vi "FIB trapezoidal mill PXIe-6124.vi"(6 "Machine Type":u8(ring) items=["Feiss", "NVision", "Jeiss"], 7 "COM port":refnum<visa-resource-name>="COM1", 8 "Milling para":T1={"X resolution"=4096, "Z resolution"=125001, "X offset (um)"=0.0, "Z offset (um)"=0.0, "X center (um)"=0.0, "Z center (um)"=0.0, "X size (um)"=250.0, "Z size (um)"=250.0, "UL-Ang"=90.0, "UR-Ang"=90.0, "Line milling time (s)"=5.0, "Z-step (nm)"=2.0, "Lines auto pause"=1, "Auto pause"=FALSE, "Mill from Bottom"=FALSE, "FIB FOV (um)"=500.0, "Auto Profile"=FALSE, "Mill start from Last"=FALSE, "FIB PID on"=FALSE, "FIB PID reset"=TRUE, "FIB PID measured"=0, "FIB PID target"=0.0, "FIB PID target slope"=0.0, "FIB PID P"=0.001, "FIB PID I"=0.01, "FIB PID D"=0.0, "Emission (uA)"=1.36, "Suppressor (V)"=50.0, "Auto reheat"=FALSE} caption="Milling Parameters" {"Suppressor (V)" step=0.1 format="%.1g"; "Emission (uA)" step=0.1 format="%.2g"; "FIB PID measured" items=["Spec.", "B.D. 1", "B.D. 2", "Mill", "Spec. +"]; "FIB PID target slope" min=-1 max=1 step=0.1; "UR-Ang" format="%.2f"; "UL-Ang" format="%.2f"; "Z offset (um)" step=0.02 format="%.3g"; "X offset (um)" step=1 format="%.3g"; "FIB FOV (um)" format="%.3g"; "Line milling time (s)" format="%.1f"; "Z center (um)" format="%#.3g"; "X center (um)" format="%#.3g"}, 9 "Options":cluster{"Flip x":bool, "Flip z":bool}={"Flip x"=TRUE, "Flip z"=TRUE}, 10 "FIB Scan Parameters":T3={"X resolution"=512, "Z resolution"=512, "X center"=0.0, "Z center"=0.0, "X size (V)"=20.0, "Z size (V)"=20.0, "Frame line rampdown ratio"=-0.1, "Scan rate (Hz)"=2000000, "Oversampling"=2} {"Z size (V)" min=0.0 max=20.0; "X size (V)" min=0.0 max=20.0; "Frame line rampdown ratio" min=-1.0 max=1.0 step=0.05 format="%.2g"; "Scan rate (Hz)" max=4000000 format="%#.6p"; "Z resolution" max=2048; "X resolution" max=2048}, 11 "HW Config":T4={"FIB X coil"="FIB/ao0", "FIB Y coil"="FIB/ao1", "Beam blank"="FIB/port0/line0", "Ext scan"="FIB/port0/line1", "Detector"="FIB/ai0", "Post #1up"="Log/ao0", "Post #1down"="Log/ao1", "Post #2up"="Log/ao2", "Post #2down"="Log/ao3"}) -> (0 "error out":errorcluster, 1 "post-pause lines":u16, 2 "Total progress":u8(slide) scale=0.0..100.0, 3 "Line progress":u8(slide) scale=0.0..100.0)   [LabVIEW 2018]
uses:
  <vilib>/DAQmx/write.llb/DAQmx Write (Analog 2D DBL NChan NSamp).vi
  <vilib>/DAQmx/write.llb/DAQmx Write (Analog 1D DBL 1Chan NSamp).vi
  <vilib>/Analysis/baseanly.llb/Mean (DBL).vi
  <vilib>/DAQmx/write.llb/DAQmx Write (Analog DBL 1Chan 1Samp).vi
  <vilib>/DAQmx/write.llb/DAQmx Write (Analog 1D DBL NChan 1Samp).vi
  <vilib>/DAQmx/create/channels.llb/DAQmx Create Channel (AO-Voltage-Basic).vi
  <vilib>/DAQmx/configure/timing.llb/DAQmx Timing (Sample Clock).vi
  <vilib>/DAQmx/miscellaneous.llb/DAQmx Fill In Error Info.vi
  <vilib>/measure/madcrms.llb/Basic Averaged DC-RMS for 1 Chan.vi
  <vilib>/Analysis/NI_AALBase.lvlib
  <vilib>/measure/NI_MAPro.lvlib
panel:
  in  "Api":refnum<k7>(container)
  out "FIB PID measured":u8
  out "FIB PID on offset":dbl
  out "FIB PID target slope":sgl
  out "FIB PID feedback mean":dbl
  out "FIB PID FB array":dbl[](array[numeric])
  out "Beam blanked":bool=TRUE
  out "FIB PID D":sgl
  out "FIB PID I":sgl
  out "FIB PID P":sgl
  out "FIB PID target":sgl
  out "FIB PID reset":bool
  out "FIB PID on":bool
  out "FIB PID feedback":dbl
  out "UR-Ang":sgl=90.0
  out "UL-Ang":sgl=90.0
  in  "FIB bit size (nm)":dbl
  out "X offset":sgl
  out "Y offset":sgl
  in  "Sweep enabled":bool
  in  "Focus (V)":dbl min=-10.0 max=10.0 step=0.1 format="%.3g"
  in  "Imbalance (V)":dbl min=-10.0 max=10.0 step=0.1 format="%.3f"
  in  "Sweep direction":bool
  in  "Angle (V)":dbl min=-10.0 max=10.0 step=0.1 format="%.3g"
  in  "Position (V)":dbl min=-10.0 max=10.0 step=0.1 format="%.3g"
  in  "Level #":u8
  in  "Sweep #":u8=1 min=1
  out "Post #2down":tag="PXI1Slot2/ao3"
  out "Post #2up":tag="PXI1Slot2/ao2"
  out "Post #1down":tag="PXI1Slot2/ao1"
  out "Post #1up":tag="PXI1Slot2/ao0"
  out "Milling mode":T2(ring)=enum."SEM + FIB"
  out "Z voltage RT":dbl
  out "Ext scan":tag="PXI1Slot4/port0/line1"
  out "FIB Y coil":tag="PXI1Slot4/ao1"
  out "FIB X coil":tag="PXI1Slot4/ao0"
  out "Mill from Bottom":bool
  out "Line Paused":bool
  in  "Resume":bool
  in  "Manual pause":bool
  out "Auto pause":bool
  out "Line milling time (s)":sgl=10.0
  out "Lines auto pause":u16=1
  out "Y size":sgl=1.0
  out "X size":sgl=1.0
  out "Y center":sgl
  out "X center":sgl
  out "Y resolution":u32=100
  out "X resolution":u32=16384
  in  "Stop":bool
  out "Beam blank":tag="PXI1Slot4/port0/line0"
  # "% of"
  # "th line"
  # "%"
  # "Direction"
  # "Start\nfrom"
  # "<"
  # "Scan coils"
  # "Flip"
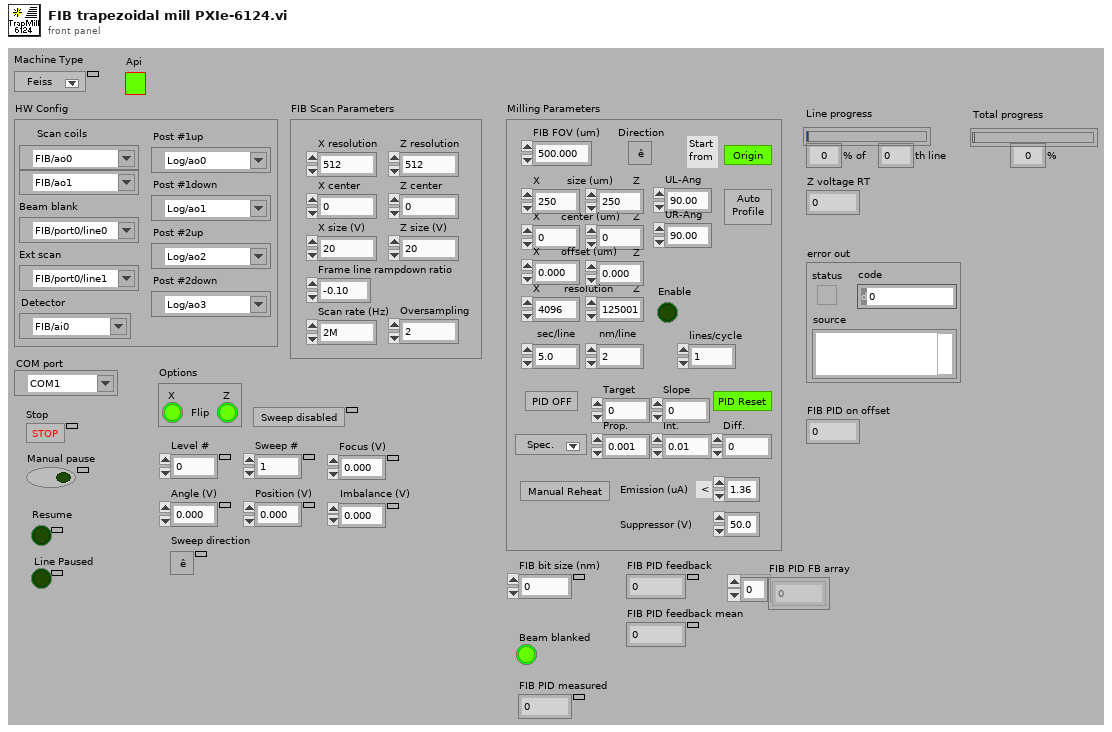
[diagram p1: front panel]
types:
  T1 = cluster{"X resolution":u32, "Z resolution":u32, "X offset (um)":sgl, "Z offset (um)":sgl, "X center (um)":sgl, "Z center (um)":sgl, "X size (um)":sgl, "Z size (um)":sgl, "UL-Ang":sgl, "UR-Ang":sgl, "Line milling time (s)":sgl, "Z-step (nm)":dbl, "Lines auto pause":u16, "Auto pause":bool, "Mill from Bottom":bool, "FIB FOV (um)":sgl, "Auto Profile":bool, "Mill start from Last":bool, "FIB PID on":bool, "FIB PID reset":bool, "FIB PID measured":u8, "FIB PID target":sgl, "FIB PID target slope":sgl, "FIB PID P":sgl, "FIB PID I":sgl, "FIB PID D":sgl, "Emission (uA)":dbl, "Suppressor (V)":sgl, "Auto reheat":bool}
  T2 = enum16{"SEM", "FIB", "Milling", "SEM + FIB", "Mill + SEM", "SEM Drift Correction", "FIB Drift Correction", "No Beam", "External", "External + SEM"}
  T3 = cluster{"X resolution":u32, "Z resolution":u32, "X center":dbl, "Z center":dbl, "X size (V)":dbl, "Z size (V)":dbl, "Frame line rampdown ratio":dbl, "Scan rate (Hz)":u32, "Oversampling":u16}
  T4 = cluster{"FIB X coil":tag, "FIB Y coil":tag, "Beam blank":tag, "Ext scan":tag, "Detector":tag, "Post #1up":tag, "Post #1down":tag, "Post #2up":tag, "Post #2down":tag}
  T5 = enum16{"SEM", "FIB", "Mill", "SEM + FIB", "Mill + SEM", "Drift SEM", "Drift FIB", "None", "Ext", "Ext + SEM"}
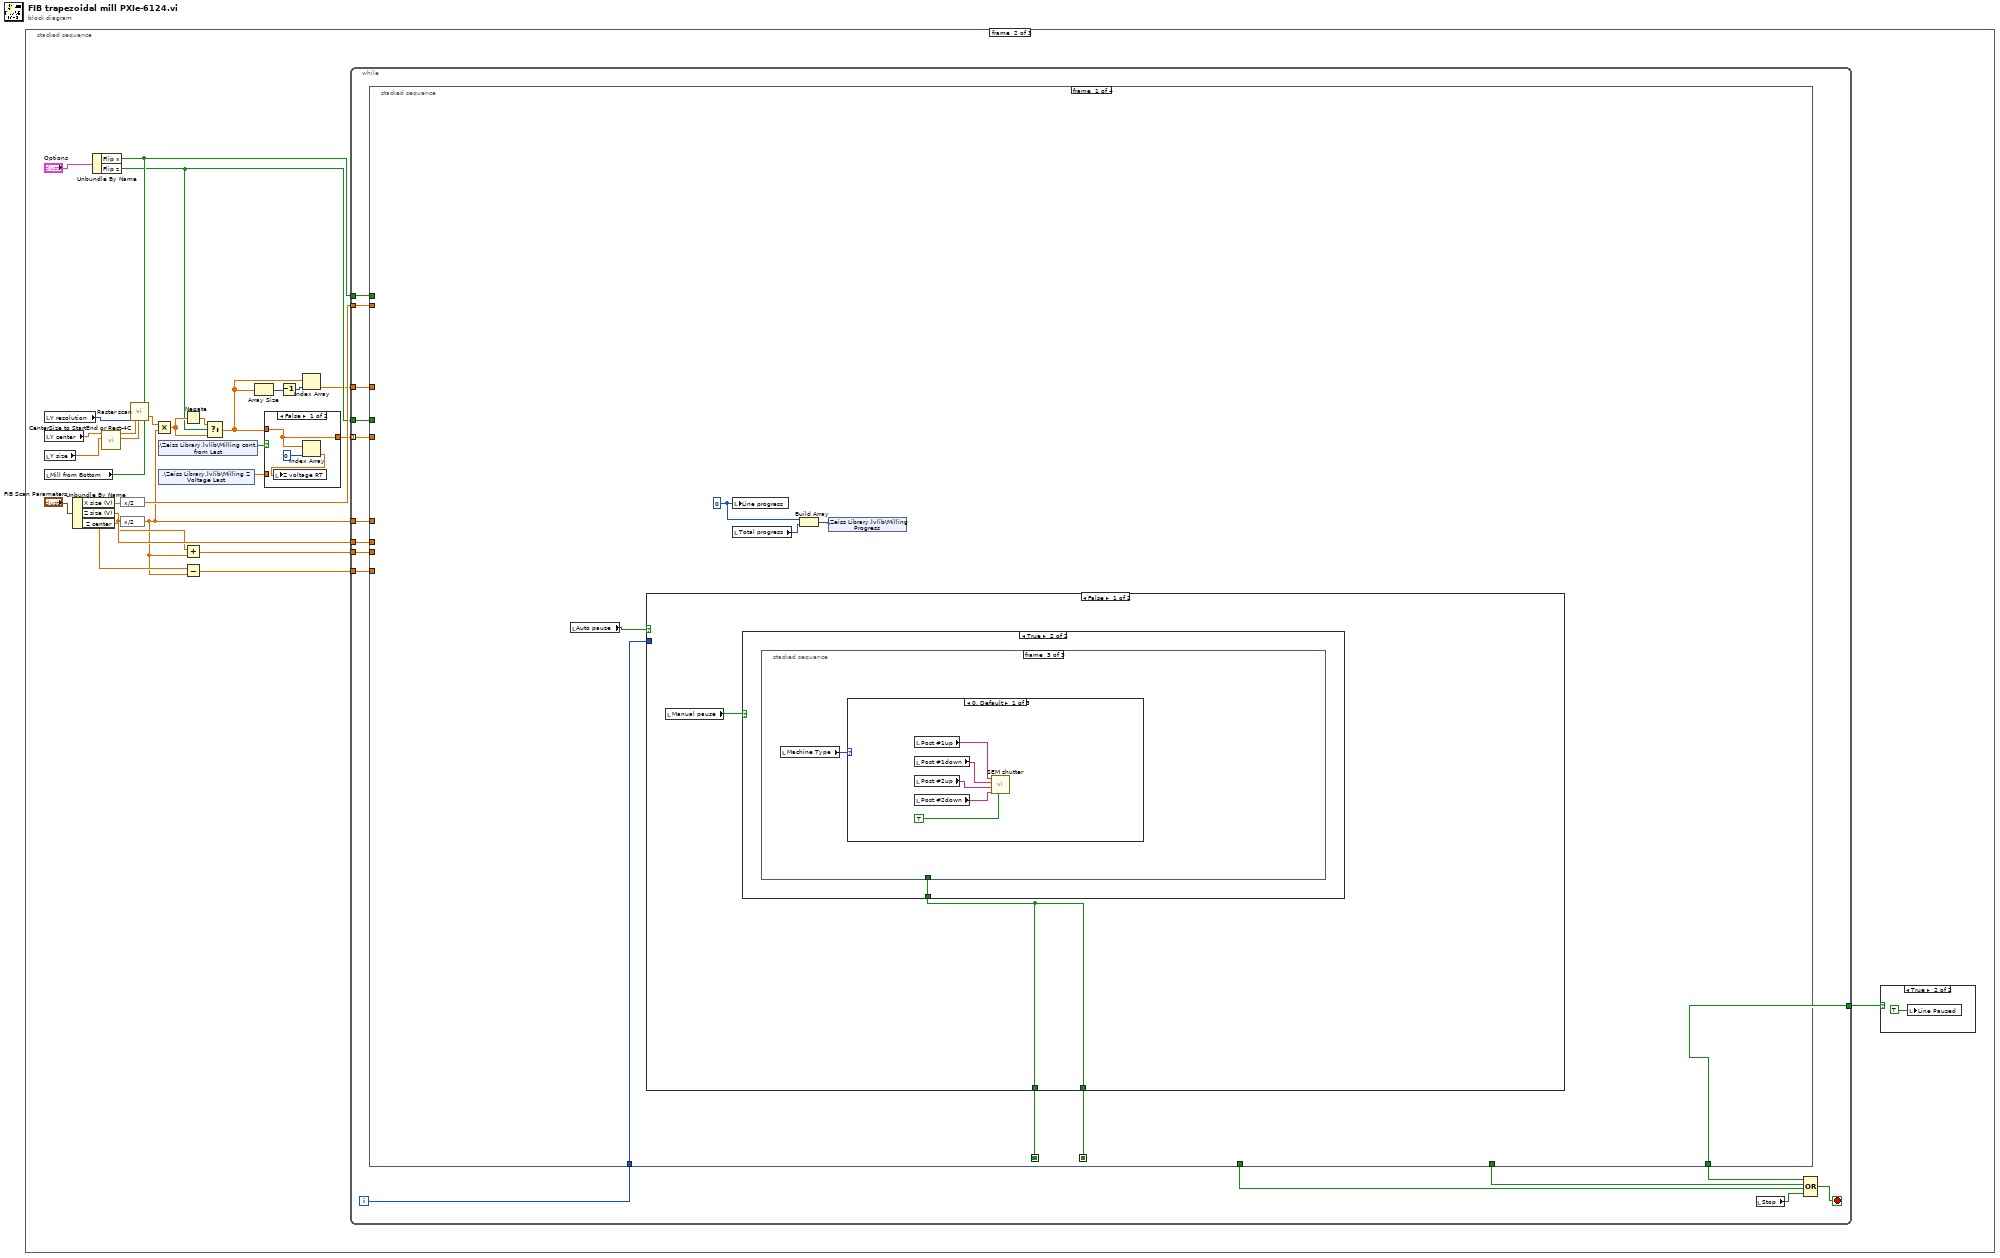
[diagram p0: block diagram]
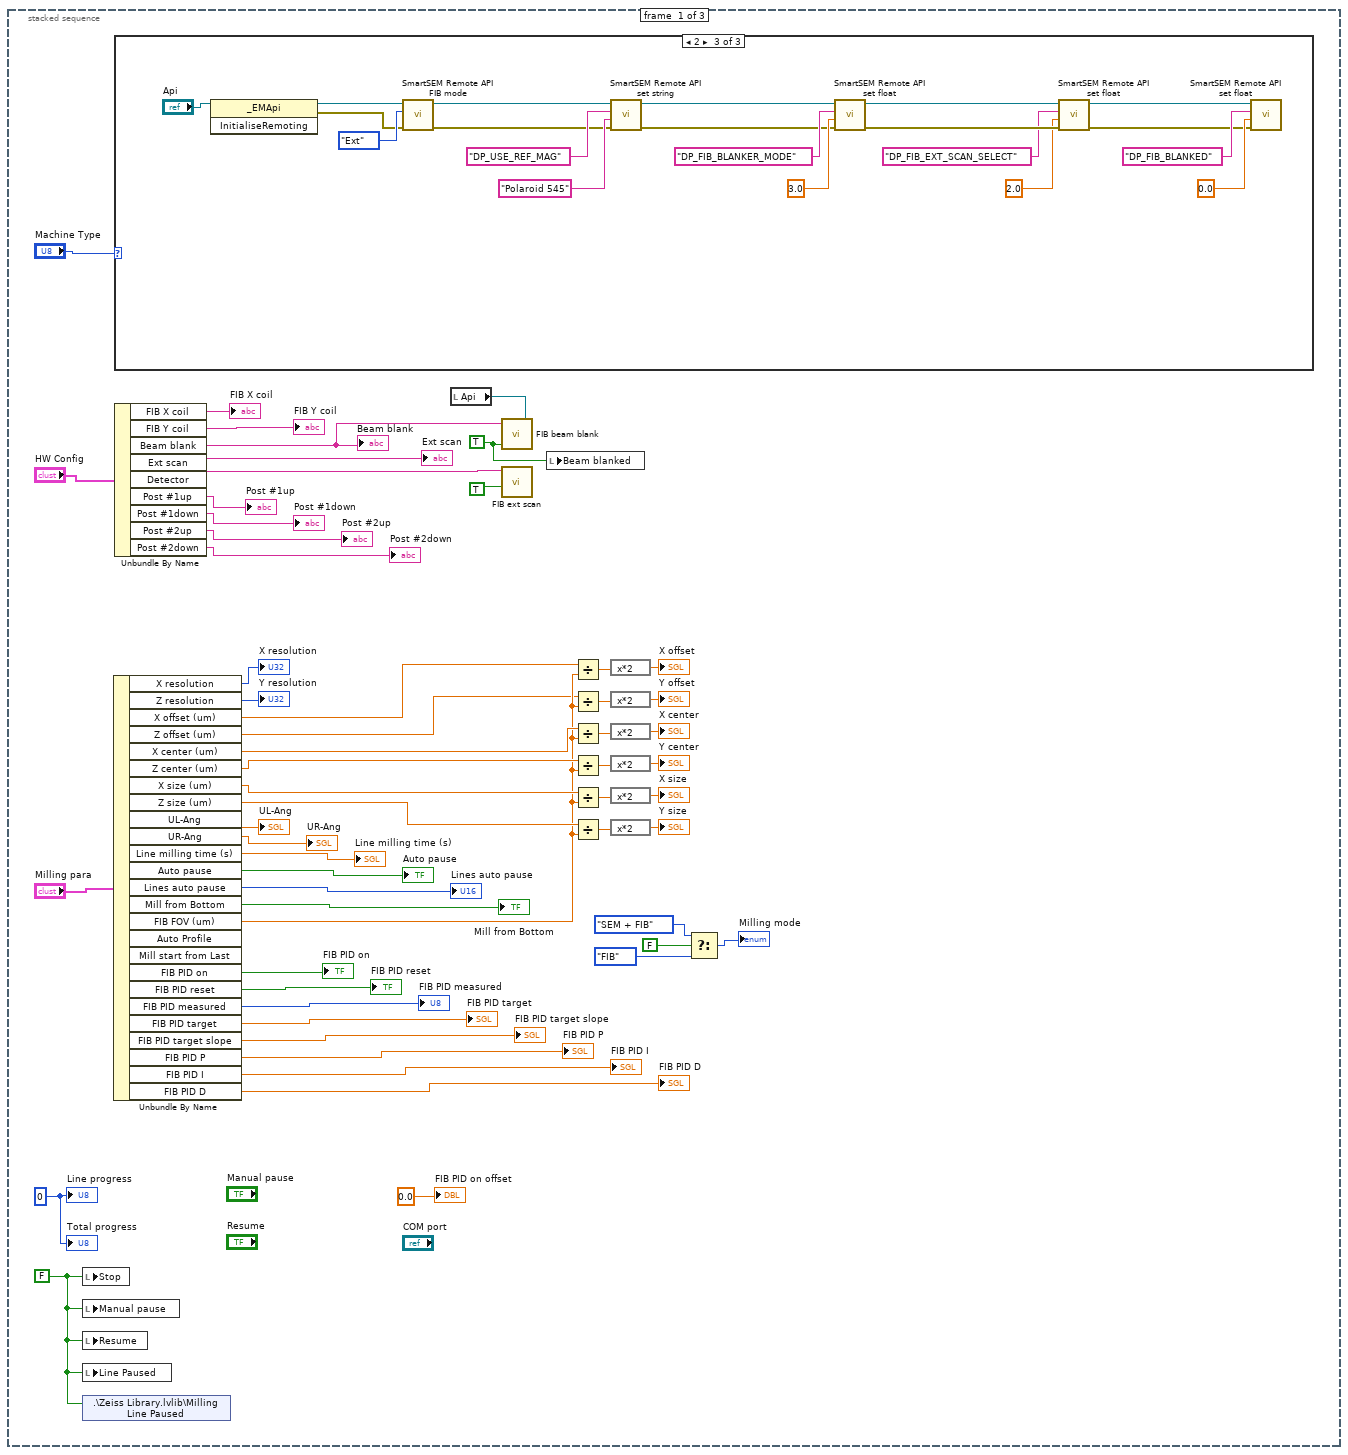
[diagram p2: hidden frame]
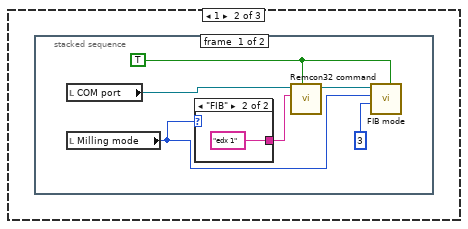
[diagram p4: hidden frame]
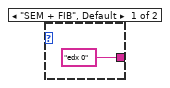
[diagram p5: hidden frame]
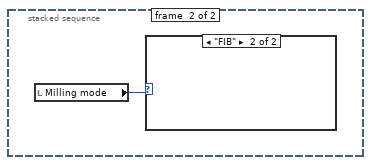
[diagram p6: hidden frame]
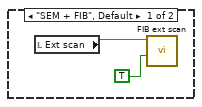
[diagram p7: hidden frame]
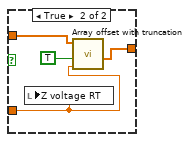
[diagram p8: hidden frame]
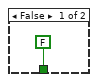
[diagram p10: hidden frame]
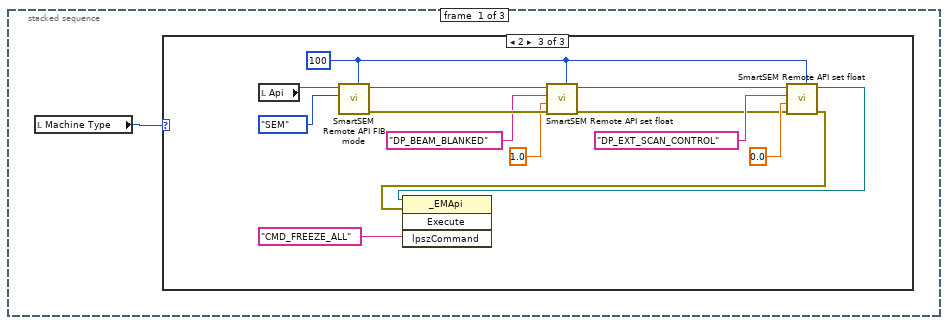
[diagram p11: hidden frame]
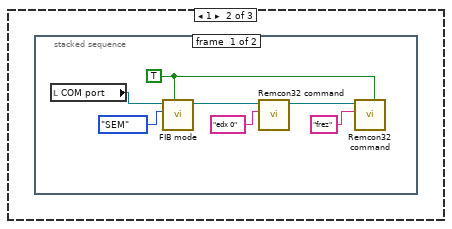
[diagram p13: hidden frame]
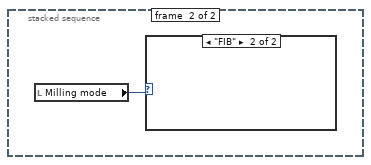
[diagram p14: hidden frame]
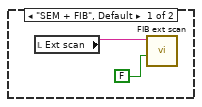
[diagram p15: hidden frame]
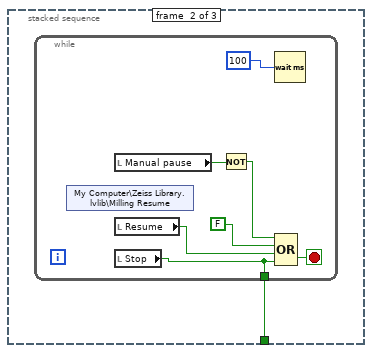
[diagram p16: hidden frame]
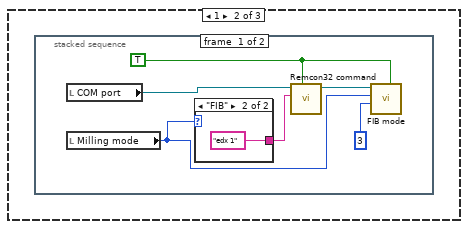
[diagram p17: hidden frame]
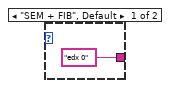
[diagram p18: hidden frame]
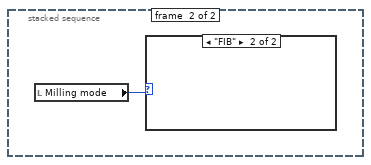
[diagram p19: hidden frame]
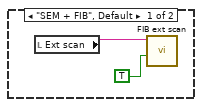
[diagram p20: hidden frame]
diagram:
  n1 = stacked-sequence {
    frame #0 {
      w7 = TRUE ("Beam blanked")
      w46 = FALSE ("Stop")
      w56 = u8 0 ("Milling progress")
      n2 = local write "Stop"(w46) -> ()
      n3 = local write "Manual pause"(w46) -> ()
      n4 = local write "Resume"(w46) -> ()
      n5 = local write "Line Paused"(w46) -> ()
      n6 = shared-variable ".\\Zeiss Library.lvlib\\Milling Line Paused"(w46) -> ()  [unwired: 1 in, 1 out]
      n7 = Unbundle By Name("Milling para") -> ("X resolution"=→"X resolution":u32, "Z resolution"=→"Y resolution":u32, "X offset (um)"=w22:sgl, "Z offset (um)"=w21:sgl, "X center (um)"=w27:sgl, "Z center (um)"=w26:sgl, "X size (um)"=w37:sgl, "Z size (um)"=w33:sgl, "UL-Ang"=→"UL-Ang":sgl, "UR-Ang"=→"UR-Ang":sgl, "Line milling time (s)"=→"Line milling time (s)":sgl, "Auto pause"=→"Auto pause":bool, "Lines auto pause"=→"Lines auto pause":u16, "Mill from Bottom"=→"Mill from Bottom":bool, "FIB FOV (um)"=w23:sgl, "FIB PID on"=→"FIB PID on":bool, "FIB PID reset"=→"FIB PID reset":bool, "FIB PID measured"=→"FIB PID measured":u8, "FIB PID target"=→"FIB PID target":sgl, "FIB PID target slope"=→"FIB PID target slope":sgl, "FIB PID P"=→"FIB PID P":sgl, "FIB PID I"=→"FIB PID I":sgl, "FIB PID D"=→"FIB PID D":sgl)  [unwired: 2 out]
      n8 = case shown="2" "Machine Type" {
        frame 0, Default {
        }
        frame 1 {
          n9 = stacked-sequence {
            frame #0 {
              w59 = TRUE ("Initialization")
              n10 = local read "COM port"() -> (w61:refnum<visa-resource-name>)
              n11 = local read "Milling mode"() -> (w57:T2)
              n12 = case shown="\"FIB\"" w57 {
                tunnel: ["edx 0" ("SEM command") "edx 1" ("SEM command")] -> w58
                frame "SEM + FIB", Default {
                }
                frame "FIB" {
                }
              }
              n13 = call "Remcon32 command.vi"("Initialization"=w59, "SEM command"=w58, "COM port in"=w61) -> ("COM port out"=w60:refnum<visa-resource-name>)  [unwired: 5 in, 3 out]
              n14 = call "FIB mode.vi"("Close session"=w59, "Iterations"=u32 3, "FIB mode"=w57, "COM port in"=w60) -> ()  [unwired: 6 in, 2 out]
            }
            frame #1 {
              n15 = local read "Milling mode"() -> (w65:T2)
              n16 = case shown="\"FIB\"" w65 {
                frame "SEM + FIB", Default {
                  n17 = local read "Ext scan"() -> (w66:tag)
                  n18 = call "FIB ext scan.vi"("Ext on"=TRUE ("data"), "FIB Ext Scan"=w66) -> ()  [unwired: 9 in, 1 out]
                }
                frame "FIB" {
                }
              }
            }
          }
        }
        frame 2 {
          n19 = invoke class="_EMApi" method="InitialiseRemoting"(reference="Api") -> (reference out=w85:refnum<k7>, error out=w84:errorcluster)  [unwired: 2 in, 1 out]
          n20 = call "SmartSEM Remote API FIB mode.vi"("error in"=w84, "FIB mode"=T5."Ext", "Api"=w85) -> ("error out"=w68:errorcluster, "Api out"=w71:refnum<k7>)  [unwired: 7 in]
          n21 = call "SmartSEM Remote API set string.vi"("error in"=w68, "vValue"="Polaroid 545" ("lpszParam"), "lpszParam"="DP_USE_REF_MAG", "Api"=w71) -> ("error out"=w69:errorcluster, "Api out"=w70:refnum<k7>)  [unwired: 6 in]
          n22 = call "SmartSEM Remote API set float.vi"("error in"=w69, "vValue"=sgl 3.0, "lpszParam"="DP_FIB_BLANKER_MODE", "Api"=w70) -> ("error out"=w78:errorcluster, "Api out"=w79:refnum<k7>)  [unwired: 6 in]
          n23 = call "SmartSEM Remote API set float.vi"("error in"=w78, "vValue"=sgl 2.0, "lpszParam"="DP_FIB_EXT_SCAN_SELECT" ("lpszCommand"), "Api"=w79) -> ("error out"=w72:errorcluster, "Api out"=w73:refnum<k7>)  [unwired: 6 in]
          n24 = call "SmartSEM Remote API set float.vi"("error in"=w72, "vValue"=sgl 0.0, "lpszParam"="DP_FIB_BLANKED", "Api"=w73) -> ()  [unwired: 6 in, 2 out]
        }
      }
      n25 = Unbundle By Name("HW Config") -> ("FIB X coil"=→"FIB X coil":tag, "FIB Y coil"=→"FIB Y coil":tag, "Beam blank"=w43:tag, "Ext scan"=w44:tag, "Post #1up"=→"Post #1up":tag, "Post #1down"=→"Post #1down":tag, "Post #2up"=→"Post #2up":tag, "Post #2down"=→"Post #2down":tag)  [unwired: 1 out]
      "Beam blank" <- w43
      "Ext scan" <- w44
      n26 = local read "Api"() -> (w2:refnum<k7>)
      n27 = call "FIB beam blank.vi"("Api"=w2, "Beam blanked"=w7, "lines"=w43) -> ()  [unwired: 2 in, 1 out]
      n28 = call "FIB ext scan.vi"("Ext on"=TRUE ("data"), "FIB Ext Scan"=w44) -> ()  [unwired: 9 in, 1 out]
      n29 = local write "Beam blanked"(w7) -> ()
      n30 = Divide(x=w22, y=w23) -> (x/y=w25:sgl)
      n31 = Divide(x=w21, y=w23) -> (x/y=w24:sgl)
      n32 = Divide(x=w27, y=w23) -> (x/y=w30:sgl)
      n33 = Divide(x=w26, y=w23) -> (x/y=w31:sgl)
      n34 = Divide(x=w37, y=w23) -> (x/y=w36:sgl)
      n35 = Divide(x=w33, y=w23) -> (x/y=w34:sgl)
      n36 = expression code="x*2"(w25) -> (→"X offset":sgl)
      n37 = expression code="x*2"(w24) -> (→"Y offset":sgl)
      n38 = expression code="x*2"(w30) -> (→"X center":sgl)
      n39 = expression code="x*2"(w31) -> (→"Y center":sgl)
      n40 = expression code="x*2"(w36) -> (→"X size":sgl)
      n41 = expression code="x*2"(w34) -> (→"Y size":sgl)
      n42 = Select(t=T2."SEM + FIB" ("FIB mode"), s=FALSE, f=T2."FIB" ("FIB mode")) -> (s? t:f=→"Milling mode":T2)
      "Line progress" <- w56
      "Total progress" <- w56
      "FIB PID on offset" <- 0.0 ("FIB PID on offset")
    }
    frame #1 {
      n43 = local read "Y resolution"() -> (w115:u32)
      n44 = local read "Y center"() -> (w114:sgl)
      n45 = local read "Y size"() -> (w107:sgl)
      n46 = local read "Mill from Bottom"() -> (w104:bool)
      n47 = Unbundle By Name("FIB Scan Parameters") -> ("X size (V)"=w108:dbl, "Z size (V)"=w101:dbl, "Z center"=w92:dbl)
      n48 = Unbundle By Name("Options") -> ("Flip x"=w103:bool, "Flip z"=w98:bool)
      n49 = call "CenterSize to StartEnd or Rect-4C.vi"("Size"=w107, "Center"=w114) -> ("End"=w112:dbl, "Start"=w113:dbl)  [unwired: 3 in, 1 out]
      n50 = expression code="x/2"(w108) -> (w102:dbl)
      n51 = expression code="x/2"(w101) -> (w91:dbl)
      n52 = call "Raster scan.vi"("Y resolution"=w115, "Y start"=w113, "Y end"=w112, "Flip x"=w103, "Flip y"=w104) -> ("Y single line pattern"=w105:dbl[])  [unwired: 7 in, 7 out]
      n53 = Multiply(x=w105, y=w91) -> (x*y=w106:dbl[])
      n54 = shared-variable ".\\Zeiss Library.lvlib\\Milling cont. from Last"() -> (w88:bool)  [unwired: 1 in, 1 out]
      n55 = shared-variable ".\\Zeiss Library.lvlib\\Milling Z Voltage Last"() -> (w99:sgl)  [unwired: 1 in, 1 out]
      n56 = Negate(x=w106) -> (-x=w110:dbl[])
      n57 = Add(x=w92, y=w91) -> (x+y=w90:dbl)
      n58 = Subtract(x=w92, y=w91) -> (x-y=w89:dbl)
      n59 = Select(t=w110, s=w98, f=w106) -> (s? t:f=w95:dbl[])
      n60 = Array Size(array=w95) -> (size(s)=w97:i32)
      n61 = case shown="False" w88 {
        tunnel: w95 -> [w118 w121]
        tunnel: [w118 w122] -> w100
        tunnel: w99 -> [_ w119]
        frame False {
          n62 = Index Array(array=w118, index=0) -> (element=w117:dbl)
          n63 = local write "Z voltage RT"(w117) -> ()
        }
        frame True {
          n64 = local write "Z voltage RT"(w119) -> ()
          n65 = call "Array offset with truncation.vi"("New starting value"=w119, "Truncate up"=TRUE, "Input array"=w121) -> ("Truncated array with new starting value"=w122:dbl[])  [unwired: 7 in, 1 out]
        }
      }
      n66 = Decrement(x=w97) -> (x-1=w96:i32)
      n67 = Index Array(array=w95, index=w96) -> (element=w94:dbl)
      n68 = while {
        tunnel: w100 -> [w133] mode=indexing
        tunnel: w103 -> [w136]
        tunnel: w102 -> [w135]
        tunnel: w91 -> [w134]
        tunnel: w101 -> [w132]
        tunnel: w98 -> [w130]
        tunnel: w94 -> [w129]
        tunnel: [w127] -> w93
        tunnel: w90 -> [w126]
        tunnel: w89 -> [w125]
        i -> [w138]
        stop <- w128 stop-if-true
        n69 = stacked-sequence {
          seq-local: [w140 _ _ _] -> [_ _ w316 _]
          seq-local: [w139 _ _ _] -> [_ _ w315 _]
          tunnel: w133 -> [_ _ w319 _]
          tunnel: w138 -> [w144 w309 _ _]
          tunnel: [_ _ w327 _] -> w131
          tunnel: [_ _ w326 _] -> w137
          tunnel: w136 -> [_ _ w321 _]
          tunnel: w135 -> [_ _ w324 _]
          tunnel: w134 -> [_ _ w325 _]
          tunnel: w132 -> [_ _ w322 _]
          tunnel: w130 -> [_ _ w323 _]
          tunnel: w129 -> [_ _ _ _]
          tunnel: [_ _ w320 _] -> w127
          tunnel: w126 -> [_ _ w318 _]
          tunnel: w125 -> [_ _ w317 _]
          frame #0 {
            w141 = u8 0 ("Line progress")
            n70 = local read "Auto pause"() -> (w145:bool)
            n71 = case shown="False" w145 {
              tunnel: w144 -> [_ w213]
              tunnel: [w146 w207] -> w140
              tunnel: [w146 w206] -> w139
              frame False {
                n72 = local read "Manual pause"() -> (w147:bool)
                n73 = case shown="True" w147 {
                  tunnel: [FALSE ("Stop") w149] -> w146
                  frame False {
                  }
                  frame True {
                    n74 = stacked-sequence {
                      tunnel: [_ w175 _] -> w149
                      frame #0 {
                        n75 = local read "Machine Type"() -> (w150:u8)
                        n76 = case shown="2" w150 {
                          frame 0, Default {
                          }
                          frame 1 {
                            n77 = stacked-sequence {
                              frame #0 {
                                w152 = TRUE ("Initialization")
                                n78 = local read "COM port"() -> (w151:refnum<visa-resource-name>)
                                n79 = call "FIB mode.vi"("Initialization"=w152, "FIB mode"=T2."SEM", "COM port in"=w151) -> ("COM port out"=w157:refnum<visa-resource-name>)  [unwired: 7 in, 1 out]
                                n80 = call "Remcon32 command.vi"("SEM command"="edx 0", "COM port in"=w157) -> ("COM port out"=w156:refnum<visa-resource-name>)  [unwired: 6 in, 3 out]
                                n81 = call "Remcon32 command.vi"("Close session"=w152, "SEM command"="frez", "COM port in"=w156) -> ()  [unwired: 5 in, 4 out]
                              }
                              frame #1 {
                                n82 = local read "Milling mode"() -> (w158:T2)
                                n83 = case shown="\"FIB\"" w158 {
                                frame "SEM + FIB", Default {
                                n84 = local read "Ext scan"() -> (w159:tag)
                                n85 = call "FIB ext scan.vi"("Ext on"=FALSE ("data"), "FIB Ext Scan"=w159) -> ()  [unwired: 9 in, 1 out]
                                }
                                frame "FIB" {
                                }
                                }
                              }
                            }
                          }
                          frame 2 {
                            w161 = u32 100 ("wait (ms)")
                            n86 = local read "Api"() -> (w172:refnum<k7>)
                            n87 = call "SmartSEM Remote API FIB mode.vi"("Wait (ms)"=w161, "FIB mode"=T5."SEM", "Api"=w172) -> ("error out"=w170:errorcluster, "Api out"=w171:refnum<k7>)  [unwired: 7 in]
                            n88 = call "SmartSEM Remote API set float.vi"("wait (ms)"=w161, "error in"=w170, "vValue"=sgl 1.0, "lpszParam"="DP_BEAM_BLANKED", "Api"=w171) -> ("error out"=w164:errorcluster, "Api out"=w165:refnum<k7>)  [unwired: 5 in]
                            n89 = call "SmartSEM Remote API set float.vi"("wait (ms)"=w161, "error in"=w164, "vValue"=sgl 0.0, "lpszParam"="DP_EXT_SCAN_CONTROL" ("lpszCommand"), "Api"=w165) -> ("error out"=w162:errorcluster, "Api out"=w163:refnum<k7>)  [unwired: 5 in]
                            n90 = invoke class="_EMApi" method="Execute"(reference=w163, error in=w162, "lpszCommand"="CMD_FREEZE_ALL") -> ()  [unwired: 1 in, 4 out]
                          }
                        }
                      }
                      frame #1 {
                        n91 = while {
                          tunnel: [w176] -> w175
                          stop <- w181 stop-if-true
                          n92 = shared-variable "My Computer\\Zeiss Library.lvlib\\Milling Resume"() -> ()  [unwired: 1 in, 2 out]
                          n93 = local read "Manual pause"() -> (w179:bool)
                          n94 = local read "Resume"() -> (w180:bool)
                          n95 = local read "Stop"() -> (w176:bool)
                          n96 = Not(x=w179) -> (.not. x?=w178:bool)
                          n97 = Wait (ms)(milliseconds to wait=u32 100) -> ()  [unwired: 1 out]
                          n98 = Compound Arithmetic op=OR(w178, FALSE ("value"), w180, w176) -> (w181:bool)
                        }
                      }
                      frame #2 {
                        n99 = local read "Machine Type"() -> (w183:u8)
                        n100 = case shown="0, Default" w183 {
                          frame 0, Default {
                            n101 = local read "Post #1up"() -> (w188:tag)
                            n102 = local read "Post #1down"() -> (w187:tag)
                            n103 = local read "Post #2up"() -> (w185:tag)
                            n104 = local read "Post #2down"() -> (w184:tag)
                            n105 = call "SEM shutter.vi"("Shutter close"=TRUE, "Shutter AO4"=w184, "Shutter AO3"=w185, "Shutter AO2"=w187, "Shutter AO1"=w188) -> ()  [unwired: 6 in, 1 out]
                          }
                          frame 1 {
                            n106 = stacked-sequence {
                              frame #0 {
                                w191 = TRUE ("Initialization")
                                n107 = local read "COM port"() -> (w193:refnum<visa-resource-name>)
                                n108 = local read "Milling mode"() -> (w189:T2)
                                n109 = case shown="\"FIB\"" w189 {
                                tunnel: ["edx 0" ("SEM command") "edx 1" ("SEM command")] -> w190
                                frame "SEM + FIB", Default {
                                }
                                frame "FIB" {
                                }
                                }
                                n110 = call "Remcon32 command.vi"("Initialization"=w191, "SEM command"=w190, "COM port in"=w193) -> ("COM port out"=w192:refnum<visa-resource-name>)  [unwired: 5 in, 3 out]
                                n111 = call "FIB mode.vi"("Close session"=w191, "Iterations"=u32 3, "FIB mode"=w189, "COM port in"=w192) -> ()  [unwired: 6 in, 2 out]
                              }
                              frame #1 {
                                n112 = local read "Milling mode"() -> (w197:T2)
                                n113 = case shown="\"FIB\"" w197 {
                                frame "SEM + FIB", Default {
                                n114 = local read "Ext scan"() -> (w198:tag)
                                n115 = call "FIB ext scan.vi"("Ext on"=TRUE ("data"), "FIB Ext Scan"=w198) -> ()  [unwired: 9 in, 1 out]
                                }
                                frame "FIB" {
                                }
                                }
                              }
                            }
                          }
                          frame 2 {
                            n116 = local read "Api"() -> (w202:refnum<k7>)
                            n117 = call "SmartSEM Remote API FIB mode.vi"("FIB mode"=T5."Ext", "Api"=w202) -> ("error out"=w200:errorcluster, "Api out"=w201:refnum<k7>)  [unwired: 8 in]
                            n118 = invoke class="_EMApi" method="Set"(reference=w201, error in=w200, "lpszParam"="DP_FIB_BLANKED", "vValue"=sgl 0.0) -> ()  [unwired: 1 in, 5 out]
                          }
                        }
                      }
                    }
                  }
                }
              }
              frame True {
                n119 = local read "Lines auto pause"() -> (w208:u16)
                n120 = Quotient & Remainder(x=w213, y=w208) -> (x-y*floor(x/y)=w214:i32, floor(x/y)=w212:i32)
                n121 = Equal To 0?(x=w214) -> (x = 0?=w210:bool)
                n122 = Not Equal To 0?(x=w212) -> (x != 0?=w211:bool)
                n123 = And(x=w210, y=w211) -> (x .and. y?=w209:bool)
                n124 = case shown="True" w209 {
                  tunnel: [w215 w218] -> w207
                  tunnel: [w215 w217] -> w206
                  frame False {
                    w215 = FALSE ("Stop")
                    n125 = local write "FIB PID reset"(TRUE ("FIB PID reset")) -> ()
                  }
                  frame True {
                    n126 = stacked-sequence {
                      tunnel: [_ w222 _ _ _ _] -> w218
                      tunnel: [_ _ _ w241 _ _] -> w217
                      frame #0 {
                        w220 = TRUE ("Beam blanked")
                        n127 = local read "Api"() -> (w219:refnum<k7>)
                        n128 = local read "Beam blank"() -> (w221:tag)
                        n129 = call "FIB beam blank.vi"("Api"=w219, "Beam blanked"=w220, "lines"=w221) -> ()  [unwired: 2 in, 1 out]
                        n130 = local write "Beam blanked"(w220) -> ()
                        "Line Paused" <- w220
                      }
                      frame #1 {
                        n131 = local read "Machine Type"() -> (w223:u8)
                        n132 = while {
                          tunnel: w223 -> [w225]
                          tunnel: [w224] -> w222
                          stop <- w226 stop-if-true
                          n133 = case shown="0, Default" w225 {
                            frame 1 {
                            }
                            frame 0, Default {
                              n134 = shared-variable ".\\Zeiss Library.lvlib\\Logs"() -> (w236:sgl[])  [unwired: 1 in, 1 out]
                              n135 = shared-variable ".\\Zeiss Library.lvlib\\Faraday cup offset"() -> (w232:sgl)  [unwired: 1 in, 1 out]
                              n136 = Index Array(array=w236, index=0) -> (element=w230:sgl)
                              n137 = Subtract(x=w230, y=w232) -> (x-y=w231:sgl)
                              n138 = Less?(x=w231, y=sgl 0.1) -> (x < y?=w233:bool)
                              n139 = case shown="True" w233 {
                                frame False {
                                }
                                frame True {
                                n140 = local read "Api"() -> (w237:refnum<k7>)
                                n141 = local read "Beam blank"() -> (w239:tag)
                                n142 = call "FIB beam blank.vi"("Api"=w237, "Beam blanked"=TRUE, "lines"=w239) -> ()  [unwired: 2 in, 1 out]
                                }
                              }
                            }
                          }
                          n143 = Wait Until Next ms Multiple(millisecond multiple=u32 100 ("milliseconds to wait")) -> ()  [unwired: 1 out]
                          n144 = shared-variable "My Computer\\Zeiss Library.lvlib\\Milling Resume"() -> (w227:bool)  [unwired: 1 in, 1 out]
                          n145 = local read "Resume"() -> (w228:bool)
                          n146 = local read "Stop"() -> (w224:bool)
                          n147 = Compound Arithmetic op=OR(w227, w228, w224) -> (w226:bool)
                        }
                      }
                      frame #2 {
                        w240 = FALSE ("Resume")
                        n148 = local write "Resume"(w240) -> ()
                        n149 = shared-variable "My Computer\\Zeiss Library.lvlib\\Milling Resume"(w240) -> ()  [unwired: 1 in, 1 out]
                        n150 = local write "Line Paused"(w240) -> ()
                      }
                      frame #3 {
                        n151 = local read "Manual pause"() -> (w242:bool)
                        n152 = case shown="True" w242 {
                          tunnel: [FALSE ("Stop") w244] -> w241
                          frame False {
                          }
                          frame True {
                            n153 = stacked-sequence {
                              seq-local: [w245 _] -> [_ w252]
                              tunnel: [w245 _] -> w244
                              frame #0 {
                                n154 = while {
                                tunnel: [w246] -> w245
                                stop <- w250 stop-if-true
                                n155 = local read "Manual pause"() -> (w248:bool)
                                n156 = Wait Until Next ms Multiple(millisecond multiple=u32 100 ("milliseconds to wait")) -> ()  [unwired: 1 out]
                                n157 = local read "Resume"() -> (w247:bool)
                                n158 = local read "Stop"() -> (w246:bool)
                                n159 = Not(x=w248) -> (.not. x?=w249:bool)
                                n160 = Compound Arithmetic op=OR(w249, w247, w246) -> (w250:bool)
                                }
                              }
                              frame #1 {
                                n161 = case shown="False" w252 {
                                frame False {
                                n162 = local read "Machine Type"() -> (w253:u8)
                                n163 = case shown="2" w253 {
                                frame 0, Default {
                                }
                                frame 1 {
                                n164 = stacked-sequence {
                                frame #0 {
                                w256 = TRUE ("Initialization")
                                n165 = local read "COM port"() -> (w258:refnum<visa-resource-name>)
                                n166 = local read "Milling mode"() -> (w254:T2)
                                n167 = case shown="\"FIB\"" w254 {
                                tunnel: ["edx 0" ("SEM command") "edx 1" ("SEM command")] -> w255
                                frame "SEM + FIB", Default {
                                }
                                frame "FIB" {
                                }
                                }
                                n168 = call "Remcon32 command.vi"("Initialization"=w256, "SEM command"=w255, "COM port in"=w258) -> ("COM port out"=w257:refnum<visa-resource-name>)  [unwired: 5 in, 3 out]
                                n169 = call "FIB mode.vi"("Close session"=w256, "Iterations"=u32 3, "FIB mode"=w254, "COM port in"=w257) -> ()  [unwired: 6 in, 2 out]
                                }
                                frame #1 {
                                n170 = local read "Milling mode"() -> (w262:T2)
                                n171 = case shown="\"SEM + FIB\", Default" w262 {
                                frame "SEM + FIB", Default {
                                n172 = local read "Ext scan"() -> (w263:tag)
                                n173 = call "FIB ext scan.vi"("Ext on"=TRUE ("data"), "FIB Ext Scan"=w263) -> ()  [unwired: 9 in, 1 out]
                                }
                                frame "FIB" {
                                }
                                }
                                }
                                }
                                }
                                frame 2 {
                                w278 = u32 100 ("wait (ms)")
                                n174 = local read "Api"() -> (w275:refnum<k7>)
                                n175 = call "SmartSEM Remote API FIB mode.vi"("Wait (ms)"=w278, "FIB mode"=T5."SEM", "Api"=w275) -> ("error out"=w273:errorcluster, "Api out"=w274:refnum<k7>)  [unwired: 7 in]
                                n176 = call "SmartSEM Remote API set float.vi"("wait (ms)"=w278, "error in"=w273, "vValue"=sgl 1.0, "lpszParam"="DP_BEAM_BLANKED", "Api"=w274) -> ("error out"=w267:errorcluster, "Api out"=w268:refnum<k7>)  [unwired: 5 in]
                                n177 = call "SmartSEM Remote API set float.vi"("wait (ms)"=w278, "error in"=w267, "vValue"=sgl 0.0, "lpszParam"="DP_EXT_SCAN_CONTROL" ("lpszCommand"), "Api"=w268) -> ("error out"=w265:errorcluster, "Api out"=w266:refnum<k7>)  [unwired: 5 in]
                                n178 = invoke class="_EMApi" method="Execute"(reference=w266, error in=w265, "lpszCommand"="CMD_FREEZE_ALL") -> ()  [unwired: 1 in, 4 out]
                                }
                                }
                                }
                                frame True {
                                }
                                }
                              }
                            }
                          }
                        }
                      }
                      frame #4 {
                        n179 = local read "Post #1up"() -> (w283:tag)
                        n180 = local read "Post #1down"() -> (w282:tag)
                        n181 = local read "Post #2up"() -> (w280:tag)
                        n182 = local read "Post #2down"() -> (w279:tag)
                        n183 = call "SEM shutter.vi"("Shutter close"=TRUE, "Shutter AO4"=w279, "Shutter AO3"=w280, "Shutter AO2"=w282, "Shutter AO1"=w283) -> ()  [unwired: 6 in, 1 out]
                      }
                      frame #5 {
                        n184 = local read "Stop"() -> (w284:bool)
                        n185 = case shown="False" w284 {
                          frame False {
                            n186 = local read "Machine Type"() -> (w285:u8)
                            n187 = case shown="2" w285 {
                              frame 0, Default {
                              }
                              frame 1 {
                                n188 = stacked-sequence {
                                frame #0 {
                                w288 = TRUE ("Initialization")
                                n189 = local read "COM port"() -> (w290:refnum<visa-resource-name>)
                                n190 = local read "Milling mode"() -> (w286:T2)
                                n191 = case shown="\"FIB\"" w286 {
                                tunnel: ["edx 0" ("SEM command") "edx 1" ("SEM command")] -> w287
                                frame "SEM + FIB", Default {
                                }
                                frame "FIB" {
                                }
                                }
                                n192 = call "Remcon32 command.vi"("Initialization"=w288, "SEM command"=w287, "COM port in"=w290) -> ("COM port out"=w289:refnum<visa-resource-name>)  [unwired: 5 in, 3 out]
                                n193 = call "FIB mode.vi"("Close session"=w288, "Iterations"=u32 3, "FIB mode"=w286, "COM port in"=w289) -> ()  [unwired: 6 in, 2 out]
                                }
                                frame #1 {
                                n194 = local read "Milling mode"() -> (w294:T2)
                                n195 = case shown="\"FIB\"" w294 {
                                frame "SEM + FIB", Default {
                                n196 = local read "Ext scan"() -> (w295:tag)
                                n197 = call "FIB ext scan.vi"("Ext on"=TRUE ("data"), "FIB Ext Scan"=w295) -> ()  [unwired: 9 in, 1 out]
                                }
                                frame "FIB" {
                                }
                                }
                                }
                                }
                              }
                              frame 2 {
                                n198 = local read "Api"() -> (w305:refnum<k7>)
                                n199 = call "SmartSEM Remote API FIB mode.vi"("FIB mode"=T5."Ext", "Api"=w305) -> ("error out"=w299:errorcluster, "Api out"=w302:refnum<k7>)  [unwired: 8 in]
                                n200 = call "SmartSEM Remote API set float.vi"("error in"=w299, "vValue"=sgl 0.0, "lpszParam"="DP_FIB_BLANKED", "Api"=w302) -> ("error out"=w300:errorcluster, "Api out"=w301:refnum<k7>)  [unwired: 6 in]
                                n201 = call "SmartSEM Remote API detectors.vi"("error in"=w300, "Det A Type"="InLens", "Api"=w301) -> ()  [unwired: 7 in, 2 out]
                              }
                            }
                          }
                          frame True {
                          }
                        }
                      }
                    }
                  }
                }
              }
            }
            n202 = local write "Line progress"(w141) -> ()
            n203 = local read "Total progress"() -> (w143:u8)
            n204 = Build Array(w141, w143) -> (w142:u8[])
            n205 = shared-variable ".\\Zeiss Library.lvlib\\Milling Progress"(w142) -> ()  [unwired: 1 in, 1 out]
          }
          frame #1 {
            n206 = local read "Machine Type"() -> (w306:u8)
            n207 = local read "Lines auto pause"() -> (w310:u16)
            n208 = case shown="2" w306 {
              frame 0, Default {
              }
              frame 2 {
                n209 = local read "Api"() -> (w312:refnum<k7>)
                n210 = shared-variable "My Computer\\Zeiss Library.lvlib\\FIB FOV (um)"() -> (w313:sgl)  [unwired: 1 in, 1 out]
                n211 = call "SmartSEM Remote API FIB mag.vi"("FIB FOV (um)"=w313, "Api"=w312) -> ()  [unwired: 8 in, 2 out]
              }
            }
            n212 = Quotient & Remainder(x=w309, y=w310) -> (x-y*floor(x/y)=w311:i32)  [unwired: 1 out]
            n213 = Increment(x=w311) -> (x+1=w308:i32)
            "post-pause lines" <- w308
            n214 = local write "FIB PID FB array"(dbl[] [] ("FIB PID FB array")) -> ()
            n215 = shared-variable ".\\Zeiss Library.lvlib\\Milling Post-pause Lines"(w308) -> ()  [unwired: 1 in, 1 out]
          }
          frame #2 {
            n216 = Or(x=w315, y=w316) -> (x .or. y?=w314:bool)
            n217 = case shown="False" w314 {
              tunnel: [w450 w761] -> w327
              tunnel: [w442 w761] -> w326
              tunnel: w325 -> [w419 _]
              tunnel: w324 -> [w399 _]
              tunnel: w323 -> [w393 _]
              tunnel: w322 -> [w391 _]
              tunnel: w321 -> [w388 _]
              tunnel: [w373 w761] -> w320
              tunnel: w319 -> [w366 _]
              tunnel: w318 -> [w364 _]
              tunnel: w317 -> [w363 _]
              frame False {
                w337 = -0.01 ("x")
                w378 = -0.1 ("x")
                w441 = 10123 items=["Finite Samples"=10178, "Continuous Samples"=10123, "Hardware Timed Single Point"=12522] ("sample mode")
                n218 = local read "Milling para"() -> (w372:T1)
                n219 = Unbundle By Name(w372) -> ("X size (um)"=w386:sgl, "FIB FOV (um)"=w361:sgl)
                n220 = local read "Z voltage RT"() -> (w369:dbl)
                n221 = local read "FIB PID on"() -> (w370:bool)
                n222 = local read "FIB PID on offset"() -> (w365:dbl)
                n223 = local read "X resolution"() -> (w398:u32)
                n224 = Add(x=w366, y=w365) -> (x+y=w367:dbl)
                n225 = local read "Machine Type"() -> (w397:u8)
                n226 = local read "FIB X coil"() -> (w444:tag)
                n227 = local read "FIB Y coil"() -> (w443:tag)
                n228 = Select(t=w369, s=w370, f=w367) -> (s? t:f=w368:dbl)
                n229 = Negate(x=w368) -> (-x=w394:dbl)
                n230 = Select(t=w394, s=w393, f=w368) -> (s? t:f=w392:dbl)
                n231 = Divide(x=w392, y=w391) -> (x/y=w389:dbl)
                n232 = Multiply(x=w361, y=w389) -> (x*y=w390:dbl)
                n233 = call "Milling parameter to trapezoidal shape.vi"("Y location (um)"=w390, "Milling para"=w372) -> ("X end"=w395:dbl, "X start"=w396:dbl, "X size (um) @ Y"=w387:dbl, "Total progress"=w375:dbl)  [unwired: 5 in, 1 out]
                n234 = call "Raster scan.vi"("X resolution"=w398, "Frame line rampdown ratio"=0.0, "X start"=w396, "X end"=w395, "Flip x"=w388) -> ("X resolution with rampdown"=w401:i32, "X single line pattern"=w404:dbl[])  [unwired: 7 in, 6 out]
                n235 = case shown="True" "Sweep enabled" {
                  tunnel: [_ w484] -> w428
                  tunnel: [_ w483] -> w427
                  frame False {
                  }
                  frame True {
                    w491 = 10123 items=["Finite Samples"=10178, "Continuous Samples"=10123, "Hardware Timed Single Point"=12522] ("sample mode")
                    n236 = local read "Line milling time (s)"() -> (w489:sgl)
                    n237 = local read "Post #1up"() -> (w480:tag)
                    n238 = call "Beam deflector.vi"("Sweep direction"="Sweep direction", "Level #"="Level #", "Imbalance (V)"="Imbalance (V)", "Position (V)"="Position (V)", "Angle (V)"="Angle (V)", "Focus (V)"="Focus (V)") -> ("All posts"=w467:dbl[][])  [unwired: 5 in]
                    n239 = call-poly <vilib>:"DAQmx Create Virtual Channel.vi"("physical channels"=w480) -> ("task out"=w481:refnum<k21>, "error out"=w478:errorcluster)  [unwired: 13 in]
                    n240 = Multiply(x="Level #", y="Sweep #") -> (x*y=w474:u8)
                    n241 = local read "Post #1down"() -> (w479:tag)
                    n242 = In Range and Coerce(upper limit=u8 255 ("lower limit"), x=w474, lower limit=u8 1) -> (coerced(x)=w475:u8)  [unwired: 1 out]
                    n243 = Divide(x=w475, y=w489) -> (x/y=w490:sgl)
                    n244 = call-poly <vilib>:"DAQmx Create Virtual Channel.vi"("task in"=w481, "physical channels"=w479, "error in"=w478) -> ("task out"=w462:refnum<k21>, "error out"=w461:errorcluster)  [unwired: 11 in]
                    n245 = local read "Post #2up"() -> (w464:tag)
                    n246 = call-poly <vilib>:"DAQmx Create Virtual Channel.vi"("task in"=w462, "physical channels"=w464, "error in"=w461) -> ("task out"=w463:refnum<k21>, "error out"=w466:errorcluster)  [unwired: 11 in]
                    n247 = local read "Post #2down"() -> (w465:tag)
                    n248 = call-poly <vilib>:"DAQmx Create Virtual Channel.vi"("task in"=w463, "physical channels"=w465, "error in"=w466) -> ("task out"=w460:refnum<k21>, "error out"=w459:errorcluster)  [unwired: 11 in]
                    n249 = call-poly <vilib>:"DAQmx Timing.vi"("task/channels in"=w460, "sample mode"=w491, "rate"=w490, "error in"=w459) -> ("task out"=w486:refnum<k21>, "error out"=w485:errorcluster)  [unwired: 3 in, 7 out]
                    n250 = call-poly <vilib>:"DAQmx Write.vi"("task/channels in"=w486, "data"=w467, "error in"=w485) -> ("task out"=w487:refnum<k21>, "error out"=w488:errorcluster)  [unwired: 1 in, 10 out]
                    n251 = call <vilib>:"DAQmx Start Task.vi"("task/channels in"=w487, "error in"=w488) -> ("task out"=w484:refnum<k21>, "error out"=w483:errorcluster)  [unwired: 12 in]
                  }
                }
                n252 = Divide(x=w387, y=w386) -> (x/y=w385:dbl)
                n253 = Multiply(x=w404, y=w399) -> (x*y=w406:dbl[])
                n254 = expression code="1e6/x"(w398) -> (w408:u32)
                n255 = Negate(x=w406) -> (-x=w405:dbl[])
                n256 = Round Toward +Infinity(x=w408) -> (ceil(x): smallest int >= x=w409:u32)
                n257 = Select(t=w405, s=w388, f=w406) -> (s? t:f=w403:dbl[])
                n258 = case shown="2" w397 {
                  tunnel: [5.0 ("minimum value") 10.0 ("minimum value") 8.0 ("minimum value")] -> w332
                  tunnel: [-5.0 ("minimum value") -10.0 ("minimum value") -8.0 ("minimum value")] -> w331
                  frame 0, Default {
                  }
                  frame 1 {
                  }
                  frame 2 {
                  }
                }
                n259 = call-poly <vilib>:"DAQmx Create Virtual Channel.vi"("maximum value"=w332, "minimum value"=w331, "physical channels"=w444) -> ("task out"=w418:refnum<k21>, "error out"=w417:errorcluster)  [unwired: 6 in, 5 out]
                n260 = call-poly <vilib>:"DAQmx Create Virtual Channel.vi"("maximum value"=w332, "minimum value"=w331, "physical channels"=w443) -> ("task out"=w416:refnum<k21>, "error out"=w415:errorcluster)  [unwired: 6 in, 5 out]
                n261 = Less Or Equal?(x=100.0, y=w375) -> (x <= y?=w373:bool)
                n262 = Divide(x=sgl 0.2, y=w361) -> (x/y=w358:sgl)
                n263 = for {
                  N: w409 -> [_]
                  tunnel: w403 -> [w454]
                  tunnel: [w454] -> w402 mode=indexing
                }
                n264 = Multiply(x=w409, y=w401) -> (x*y=w410:u32)
                n265 = Random Number (0-1)() -> (number: 0 to 1=w359:dbl)
                n266 = local read "Milling para"() -> (w381:T1)
                n267 = local read "Options"() -> (w382:cluster{"Flip x":bool, "Flip z":bool})
                n268 = Reshape Array(w402, w410) -> (w407:dbl[])
                n269 = Multiply(x=w359, y=w358) -> (x*y=w357:dbl)
                n270 = local read "X offset"() -> (w356:sgl)
                n271 = local read "Y offset"() -> (w421:sgl)
                n272 = Round Toward -Infinity(1:w375) -> (0:w376:dbl)
                n273 = Add(x=w357, y=w356) -> (x+y=w355:dbl)
                n274 = Unbundle By Name(w381) -> ("Mill from Bottom"=w383:bool)
                n275 = Unbundle By Name(w382) -> ("Flip z"=w384:bool)
                n276 = Multiply(x=w355, y=w399) -> (x*y=w422:dbl)
                n277 = Multiply(x=w421, y=w419) -> (x*y=w420:dbl)
                n278 = call-poly <vilib>:"DAQmx Timing.vi"("task/channels in"=w418, "sample mode"=w441, "rate"=1000000.0 ("Milling rate"), "error in"=w417) -> ("task out"=w436:refnum<k21>, "error out"=w435:errorcluster)  [unwired: 3 in, 7 out]
                n279 = To Unsigned Byte Integer(number=w376) -> (unsigned 8bit integer=w377:u8)
                n280 = shared-variable ".\\Zeiss Library.lvlib\\Faraday Cup before mill"() -> (w329:sgl)  [unwired: 1 in, 1 out]
                n281 = Negate(x=w422) -> (-x=w423:dbl)
                n282 = Negate(x=w420) -> (-x=w425:dbl)
                n283 = Select(t=w423, s=w388, f=w422) -> (s? t:f=w424:dbl)
                n284 = Select(t=w425, s=w393, f=w420) -> (s? t:f=w371:dbl)
                n285 = Exclusive Or(1:w384, 2:w383) -> (0:w335:bool)
                n286 = Compound Arithmetic op=ADD(w424, w407) -> (w333:dbl[])
                n287 = In Range and Coerce(upper limit=w332, x=w333, lower limit=w331) -> (coerced(x)=w330:dbl[])  [unwired: 1 out]
                n288 = Add(x=w368, y=w371) -> (x+y=w411:dbl)
                n289 = call-poly <vilib>:"DAQmx Write.vi"("task/channels in"=w436, "data"=w330, "error in"=w435) -> ("task out"=w434:refnum<k21>, "error out"=w433:errorcluster)  [unwired: 1 in, 10 out]
                n290 = Negate(x=w378) -> (-x=w379:dbl)
                n291 = Negate(x=w337) -> (-x=w336:dbl)
                n292 = expression code="x/20"(w329) -> (w328:sgl)
                n293 = Select(t=w379, s=w335, f=w378) -> (s? t:f=w380:dbl)
                n294 = Select(t=w336, s=w335, f=w337) -> (s? t:f=w334:dbl)
                n295 = call <vilib>:"DAQmx Start Task.vi"("task/channels in"=w434, "error in"=w433) -> ("task out"=w432:refnum<k21>, "error out"=w431:errorcluster)  [unwired: 12 in]
                n296 = while {
                  shift-right: [w595] -> _
                  shift-left: 0.0 -> [w599]
                  shift-right: [w594] -> _
                  shift-left: _ -> [w593]
                  tunnel: [w589] -> w447
                  shift-right: [w503] -> _
                  shift-left: FALSE ("Manual pause") -> [w588]
                  tunnel: [w585] -> w440
                  tunnel: [w584] -> w446
                  tunnel: [w583] -> w445
                  tunnel: ["Stop"] -> w450
                  tunnel: w432 -> [w570]
                  tunnel: w431 -> [w569]
                  tunnel: [w546] -> w442
                  tunnel: [w575] -> w439
                  tunnel: [w566] -> w430
                  tunnel: [w565] -> w429
                  tunnel: w428 -> [w564]
                  tunnel: w427 -> [w563]
                  tunnel: "Sweep enabled" -> [w562]
                  tunnel: w416 -> [w561]
                  tunnel: w415 -> [w549]
                  tunnel: [w560] -> w414
                  tunnel: [w545] -> w413
                  tunnel: w411 -> [w553]
                  tunnel: w391 -> [w552]
                  tunnel: w385 -> [w543]
                  tunnel: w380 -> [w510]
                  tunnel: w377 -> [w524]
                  tunnel: w366 -> [w522]
                  tunnel: w364 -> [w520]
                  tunnel: w363 -> [w519]
                  shift-right: [w514] -> w352
                  shift-left: sgl[][] [] -> [w513]
                  tunnel: w334 -> [w508]
                  tunnel: w329 -> [w502]
                  tunnel: w328 -> [w501]
                  i -> [w507]
                  stop <- w596 stop-if-true
                  w574 = u32 0 ("milliseconds to wait")
                  w579 = 100.0 ("x")
                  n297 = Random Number (0-1)() -> (number: 0 to 1=w554:dbl)
                  n298 = Greater?(x=w507, y=u32 1 ("millisecond multiple")) -> (0:w505:bool)
                  n299 = local read "Line progress"() -> (w587:u8)
                  n300 = local write "Total progress"(w524) -> ()
                  n301 = local read "Manual pause"() -> (w503:bool)
                  n302 = local read "Milling para"() -> (w555:T1)
                  n303 = local read "FIB PID on"() -> (w540:bool)
                  n304 = local read "Beam blanked"() -> (w539:bool)
                  n305 = local read "Manual pause"() -> (w517:bool)
                  n306 = local read "FIB PID measured"() -> (w518:u8)
                  n307 = local read "Manual pause"() -> (w582:bool)
                  n308 = Equal To 0?(x=w507) -> (x = 0?=w542:bool)
                  n309 = Tick Count (ms)() -> (millisecond timer value=w594:u32)
                  n310 = local read "Line milling time (s)"() -> (w591:sgl)
                  n311 = Subtract(x=w594, y=w593) -> (x-y=w536:u32)
                  n312 = Wait Until Next ms Multiple(millisecond multiple=u32 100) -> ()  [unwired: 1 out]
                  n313 = expression code="x/1000"("FIB bit size (nm)") -> (w558:dbl)
                  n314 = Unbundle By Name(w555) -> ("FIB FOV (um)"=w556:sgl)
                  n315 = expression code="x*2-1"(w554) -> (w551:dbl)
                  n316 = Not(x=w539) -> (.not. x?=w538:bool)
                  n317 = Not(x=w517) -> (.not. x?=w516:bool)
                  n318 = Select(t=w510, s=w505, f=w508) -> (s? t:f=w509:dbl)
                  n319 = Build Array(w587, w524) -> (w586:u8[])
                  n320 = local read "FIB PID reset"() -> (w526:bool)
                  n321 = Compound Arithmetic op=OR(w582, w542) -> (w592:bool)
                  n322 = Not Equal?(x=w503, y=w588) -> (x != y?=w541:bool)
                  n323 = Compound Arithmetic op=AND(w540, w538, w516) -> (w523:bool)
                  n324 = shared-variable ".\\Zeiss Library.lvlib\\Milling Progress"(w586) -> ()  [unwired: 1 in, 1 out]
                  n325 = Select(t=u32 0, s=w592, f=w536) -> (s? t:f=w597:u32)
                  n326 = Compound Arithmetic op=MULTIPLY(w591, 1000.0 ("y"), w543) -> (w573:dbl)
                  n327 = Not(x=w503) -> (.not. x?=w525:bool)
                  n328 = Divide(x=w558, y=w556) -> (x/y=w559:dbl)
                  n329 = Add(x=w573, y=w574) -> (x+y=w572:dbl)
                  n330 = Add(x=w597, y=w599) -> (x+y=w595:dbl)
                  n331 = local read "Machine Type"() -> (w504:u8)
                  n332 = Compound Arithmetic op=MULTIPLY(w559, w551, w552) -> (w550:dbl)
                  n333 = local read "FIB PID target"() -> (w527:sgl)
                  n334 = local read "FIB PID target slope"() -> (w532:sgl)
                  n335 = Divide(x=w536, y=u32 1000) -> (x/y=w537:dbl)
                  n336 = Divide(x=w595, y=w572) -> (x/y=w533:dbl)
                  n337 = Greater Or Equal?(x=w595, y=w572) -> (x >= y?=w576:bool)
                  n338 = And(x=w525, y=w526) -> (x .and. y?=w515:bool)
                  n339 = expression code="(x-0.5)*2"(w533) -> (w531:dbl)
                  n340 = local read "Api"() -> (w571:refnum<k7>)
                  n341 = case shown="True" w542 {
                    tunnel: [_ w712] -> w585
                    tunnel: w574 -> [_ w711]
                    tunnel: w571 -> [_ w710]
                    frame False {
                    }
                    frame True {
                      n342 = stacked-sequence {
                        tunnel: [_ w717] -> w712
                        tunnel: w711 -> [w713 _]
                        tunnel: w710 -> [_ w714]
                        frame #0 {
                          n343 = Wait (ms)(milliseconds to wait=w713) -> ()  [unwired: 1 out]
                        }
                        frame #1 {
                          w715 = FALSE ("Beam blanked")
                          n344 = local read "Beam blank"() -> (w716:tag)
                          n345 = local write "Beam blanked"(w715) -> ()
                          n346 = call "FIB beam blank.vi"("Api"=w714, "Beam blanked"=w715, "lines"=w716) -> ("error out"=w717:errorcluster)  [unwired: 2 in]
                        }
                      }
                    }
                  }
                  n347 = Sign(1:w527) -> (0:w499:sgl)
                  n348 = Multiply(x=-1.0, y=w499) -> (x*y=w498:dbl)
                  n349 = case shown="True" w541 {
                    tunnel: [_ w720] -> w589
                    tunnel: w503 -> [_ w719]
                    tunnel: w504 -> [_ w718]
                    frame False {
                    }
                    frame True {
                      n350 = case shown="False" w719 {
                        tunnel: [w722 w756] -> w720
                        tunnel: w718 -> [w721 w754]
                        frame False {
                          n351 = stacked-sequence {
                            tunnel: [_ _ _ _ _ w751] -> w722
                            tunnel: w721 -> [w723 w736 _ _ _ _]
                            frame #0 {
                              n352 = case shown="0, Default" w723 {
                                frame 0, Default {
                                }
                                frame 1 {
                                w726 = TRUE ("Initialization")
                                n353 = local read "COM port"() -> (w727:refnum<visa-resource-name>)
                                n354 = local read "Milling mode"() -> (w725:T2)
                                n355 = case shown="\"FIB\"" w725 {
                                tunnel: ["edx 0" ("SEM command") "edx 1" ("SEM command")] -> w724
                                frame "SEM + FIB", Default {
                                }
                                frame "FIB" {
                                }
                                }
                                n356 = call "Remcon32 command.vi"("Close session"=w726, "Initialization"=w726, "SEM command"=w724, "COM port in"=w727) -> ()  [unwired: 4 in, 4 out]
                                }
                                frame 2 {
                                n357 = local read "Api"() -> (w734:refnum<k7>)
                                n358 = call "SmartSEM Remote API FIB mode.vi"("FIB mode"=T5."Ext", "Api"=w734) -> ("error out"=w730:errorcluster, "Api out"=w731:refnum<k7>)  [unwired: 8 in]
                                n359 = invoke class="_EMApi" method="Set"(reference=w731, error in=w730, "lpszParam"="DP_FIB_BLANKED", "vValue"=sgl 0.0) -> ()  [unwired: 1 in, 5 out]
                                }
                              }
                            }
                            frame #1 {
                              n360 = case shown="1" w736 {
                                frame 0, Default {
                                }
                                frame 1 {
                                w738 = TRUE ("Initialization")
                                n361 = local read "COM port"() -> (w739:refnum<visa-resource-name>)
                                n362 = local read "Milling mode"() -> (w737:T2)
                                n363 = call "FIB mode.vi"("Close session"=w738, "Initialization"=w738, "FIB mode"=w737, "COM port in"=w739) -> ()  [unwired: 6 in, 2 out]
                                }
                              }
                            }
                            frame #2 {
                              n364 = local read "Post #1up"() -> (w743:tag)
                              n365 = local read "Post #1down"() -> (w744:tag)
                              n366 = local read "Post #2up"() -> (w741:tag)
                              n367 = local read "Post #2down"() -> (w740:tag)
                              n368 = call "SEM shutter.vi"("Shutter close"=TRUE, "Shutter AO4"=w740, "Shutter AO3"=w741, "Shutter AO2"=w744, "Shutter AO1"=w743) -> ()  [unwired: 6 in, 1 out]
                              n369 = Wait (ms)(milliseconds to wait=u32 100) -> ()  [unwired: 1 out]
                            }
                            frame #3 {
                              n370 = local read "Ext scan"() -> (w747:tag)
                              n371 = call "FIB ext scan.vi"("Ext on"=TRUE, "FIB Ext Scan"=w747) -> ()  [unwired: 9 in, 1 out]
                            }
                            frame #4 {
                              n372 = Wait (ms)(milliseconds to wait=u32 100) -> ()  [unwired: 1 out]
                            }
                            frame #5 {
                              w750 = FALSE ("Beam blanked")
                              n373 = local read "Api"() -> (w749:refnum<k7>)
                              n374 = local read "Beam blank"() -> (w752:tag)
                              n375 = local write "Beam blanked"(w750) -> ()
                              n376 = call "FIB beam blank.vi"("Api"=w749, "Beam blanked"=w750, "lines"=w752) -> ("error out"=w751:errorcluster)  [unwired: 2 in]
                            }
                          }
                        }
                        frame True {
                          w755 = TRUE ("Beam blanked")
                          n377 = local read "Api"() -> (w753:refnum<k7>)
                          n378 = local read "Beam blank"() -> (w757:tag)
                          n379 = case shown="1" w754 {
                            frame 0, Default {
                            }
                            frame 1 {
                              w758 = TRUE ("Initialization")
                              n380 = local read "COM port"() -> (w760:refnum<visa-resource-name>)
                              n381 = call "Remcon32 command.vi"("Close session"=w758, "Initialization"=w758, "SEM command"="edx 0", "COM port in"=w760) -> ()  [unwired: 4 in, 4 out]
                            }
                            frame 2 {
                            }
                          }
                          n382 = call "FIB beam blank.vi"("Api"=w753, "Beam blanked"=w755, "lines"=w757) -> ("error out"=w756:errorcluster)  [unwired: 2 in]
                          "Beam blanked" <- w755
                        }
                      }
                    }
                  }
                  n383 = local read "Beam blanked"() -> (w511:bool)
                  n384 = call <vilib>:"DAQmx Is Task Done.vi"("task/channels in"=w570, "error in"=w569) -> ("task out"=w584:refnum<k21>, "error out"=w583:errorcluster)  [unwired: 2 in, 10 out]
                  n385 = Compound Arithmetic op=MULTIPLY(w499, w532, w531) -> (w530:dbl)
                  n386 = Increment(x=w530) -> (x+1=w529:dbl)
                  n387 = Multiply(x=w527, y=w529) -> (x*y=w528:dbl)
                  n388 = case shown="True" w523 {
                    tunnel: w537 -> [_ w619]
                    tunnel: [0.0 ("Feedback") w618] -> w544
                    tunnel: w509 -> [_ w617]
                    tunnel: w528 -> [_ w616]
                    tunnel: w518 -> [_ w615]
                    tunnel: w515 -> [_ w614]
                    tunnel: w502 -> [_ w613]
                    tunnel: w501 -> [_ w612]
                    tunnel: w498 -> [_ w611]
                    frame False {
                      n389 = local write "FIB PID FB array"(dbl[] [] ("array")) -> ()
                    }
                    frame True {
                      n390 = stacked-sequence {
                        tunnel: w619 -> [_ w654 _]
                        tunnel: [_ w650 _] -> w618
                        tunnel: w617 -> [_ w646 _]
                        tunnel: w616 -> [_ w628 _]
                        tunnel: w615 -> [_ w642 _]
                        tunnel: w614 -> [w620 _ w690]
                        tunnel: w613 -> [_ w626 _]
                        tunnel: w612 -> [_ w625 _]
                        tunnel: w611 -> [_ w624 _]
                        frame #0 {
                          n391 = case shown="True" w620 {
                            frame False {
                            }
                            frame True {
                              w621 = 0.0 ("FIB PID feedback")
                              n392 = local write "FIB PID feedback"(w621) -> ()
                              n393 = local write "FIB PID feedback mean"(w621) -> ()
                            }
                          }
                        }
                        frame #1 {
                          (unwired) 0.5 ("Measured upper limit")
                          n394 = local read "FIB PID I"() -> (w637:sgl)
                          n395 = local read "FIB PID P"() -> (w640:sgl)
                          n396 = shared-variable ".\\Zeiss Library.lvlib\\Logs"() -> (w651:sgl[])  [unwired: 1 in, 1 out]
                          n397 = case shown="0, Default" w642 {
                            tunnel: [w660 100.0 ("Measured upper limit") 100.0 ("Measured upper limit") 100.0 ("Measured upper limit") 100.0 ("Measured upper limit")] -> w643
                            tunnel: [1 ("index") 2 ("index") 3 ("index") 4 ("index") 4 ("index")] -> w635
                            tunnel: [w655 1.0 ("Measured upper limit") -1.0 ("Measured upper limit") -1.0 ("Measured upper limit") -1.0 ("Measured upper limit")] -> w638
                            tunnel: [500.0 ("Measured upper limit") 0.1 ("Measured upper limit") 500.0 ("Measured upper limit") 0.1 ("Measured upper limit") 0.1 ("Measured upper limit")] -> w631
                            tunnel: w628 -> [w659 w664 w669 w677 _]
                            tunnel: [w659 w664 w669 w676 w685] -> w627
                            tunnel: w626 -> [w657 _ _ w675 w684]
                            tunnel: w624 -> [w655 _ _ _ _]
                            frame 0, Default {
                              n398 = expression code="x/2"(w657) -> (w656:sgl)
                              n399 = Greater Than 0?(x=w659) -> (x > 0?=w658:bool)
                              n400 = Select(t=500.0 ("Measured upper limit"), s=w658, f=w656) -> (s? t:f=w660:dbl)
                            }
                            frame 1 {
                            }
                            frame 2 {
                            }
                            frame 3 {
                              n401 = In Range and Coerce(upper limit=w675, x=w677, lower limit=0.0 ("Measured upper limit")) -> (coerced(x)=w676:dbl)  [unwired: 1 out]
                            }
                            frame 4 {
                              n402 = shared-variable ".\\Zeiss Library.lvlib\\FIB mill target by spec. I"() -> (w683:sgl)  [unwired: 1 in, 1 out]
                              n403 = In Range and Coerce(upper limit=w684, x=w683, lower limit=0.0 ("Measured upper limit")) -> (coerced(x)=w685:dbl)  [unwired: 1 out]
                            }
                          }
                          n404 = Index Array(array=w651, index #1=2 ("index"), index #2=w635) -> (element #1=w633:sgl, element #2=w636:sgl)
                          n405 = Multiply(x=w637, y=w638) -> (x*y=w639:dbl)
                          n406 = Multiply(x=w640, y=w638) -> (x*y=w641:dbl)
                          n407 = Greater?(x=w633, y=w625) -> (0:w632:bool)
                          n408 = local read "FIB PID FB array"() -> (w622:dbl[])
                          n409 = Select(t=-100.0 ("Measured upper limit"), s=w632, f=w631) -> (s? t:f=w630:dbl)
                          n410 = Array Size(array=w622) -> (size(s)=w623:i32)
                          n411 = call "PID Feedback.vi"("Measured"=w636, "Proportional"=w641, "Integral"=w639, "Measured upper limit"=w643, "Measured lower limit"=w630, "Target"=w627, "Feedback offset if measured exceed limits"=w646, "Cycle time"=w654, "Feedback low limit"=-1.0 ("Low limit"), "Feedback high limit"=1.0 ("High limit")) -> ("Feedback"=w650:dbl)  [unwired: 4 in, 1 out]
                          "FIB PID feedback" <- w650
                          n412 = Build Array (concatenate)(w622, w650) -> (w645:dbl[])
                          "FIB PID FB array" <- w645
                          n413 = expression code="x-4"(w623) -> (w644:i32)
                          n414 = Array Subset(array=w645, index=4, length=w644) -> (w648:dbl[])
                          n415 = call-poly <vilib>:"Mean.vi"("X"=w648) -> ("mean"=→"FIB PID feedback mean":dbl)  [unwired: 1 out]
                        }
                        frame #2 {
                          n416 = case shown="True" w690 {
                            frame False {
                            }
                            frame True {
                              n417 = local write "FIB PID reset"(FALSE ("FIB PID reset")) -> ()
                            }
                          }
                        }
                      }
                    }
                  }
                  n418 = Compound Arithmetic op=ADD(w550, w553, w544) -> (w521:dbl)
                  n419 = In Range and Coerce(upper limit=w520, x=w521, lower limit=w519) -> (coerced(x)=w512:dbl)  [unwired: 1 out]
                  "Z voltage RT" <- w512
                  n420 = case shown="False" w511 {
                    tunnel: [w602 w605] -> w514
                    tunnel: w513 -> [w601 w605]
                    tunnel: w512 -> [w600 _]
                    frame False {
                      n421 = shared-variable ".\\Zeiss Library.lvlib\\Logs"() -> (w603:sgl[])  [unwired: 1 in, 1 out]
                      n422 = Build Array (concatenate)(w603, w600) -> (w604:dbl[])
                      n423 = Build Array (concatenate)(w601, w604) -> (w602:dbl[][])
                    }
                    frame True {
                    }
                  }
                  n424 = case shown="True" w562 {
                    tunnel: [FALSE ("status") w699] -> w567
                    tunnel: [w694 w698] -> w566
                    tunnel: [w693 w697] -> w565
                    tunnel: w564 -> [w694 w696]
                    tunnel: w563 -> [w693 w695]
                    frame False {
                    }
                    frame True {
                      n425 = call <vilib>:"DAQmx Is Task Done.vi"("task/channels in"=w696, "error in"=w695) -> ("task out"=w698:refnum<k21>, "error out"=w697:errorcluster)  [unwired: 2 in, 10 out]
                      n426 = Unbundle By Name(w697) -> ("status"=w699:bool)
                    }
                  }
                  n427 = shared-variable ".\\Zeiss Library.lvlib\\Milling Z Voltage RT"(w512) -> ()  [unwired: 1 in, 1 out]
                  n428 = case shown="True" w576 {
                    tunnel: [_ w703] -> w575
                    tunnel: [FALSE ("Beam blanked") w702] -> w568
                    tunnel: w571 -> [_ w701]
                    frame False {
                    }
                    frame True {
                      n429 = stacked-sequence {
                        tunnel: [w707 _ _] -> w703
                        tunnel: [_ _ TRUE ("Beam blanked")] -> w702
                        tunnel: w701 -> [w704 _ _]
                        frame #0 {
                          w705 = TRUE ("Beam blanked")
                          n430 = local read "Beam blank"() -> (w706:tag)
                          n431 = local write "Beam blanked"(w705) -> ()
                          n432 = call "FIB beam blank.vi"("Api"=w704, "Beam blanked"=w705, "lines"=w706) -> ("error out"=w707:errorcluster)  [unwired: 2 in]
                        }
                        frame #1 {
                          n433 = Wait (ms)(milliseconds to wait=u32 10) -> ()  [unwired: 1 out]
                        }
                        frame #2 {
                        }
                      }
                    }
                  }
                  n434 = Multiply(x=w579, y=w533) -> (x*y=w580:dbl)
                  n435 = In Range and Coerce(upper limit=w579, x=w580, lower limit=0.0) -> (coerced(x)=w578:dbl)  [unwired: 1 out]
                  n436 = local write "Line progress"(w578) -> ()
                  n437 = call-poly <vilib>:"DAQmx Write.vi"("task/channels in"=w561, "data"=w512, "error in"=w549) -> ("task out"=w560:refnum<k21>, "error out"=w545:errorcluster)  [unwired: 1 in, 10 out]
                  n438 = case shown="True" w523 {
                    tunnel: w512 -> [_ w608]
                    tunnel: w522 -> [_ w607]
                    frame False {
                    }
                    frame True {
                      n439 = Subtract(x=w608, y=w607) -> (x-y=w606:dbl)
                      n440 = local write "FIB PID on offset"(w606) -> ()
                    }
                  }
                  n441 = Unbundle By Name(w583) -> ("status"=w548:bool)
                  n442 = Unbundle By Name(w545) -> ("status"=w547:bool)
                  n443 = Or(x=w548, y=w547) -> (x .or. y?=w546:bool)
                  n444 = Compound Arithmetic op=OR(w568, w567, w546, "Stop") -> (w596:bool)
                }
                n445 = call <vilib>:"DAQmx Clear Task.vi"("task in"=w446, "error in"=w445) -> ("error out"=w449:errorcluster)  [unwired: 13 out]
                n446 = call <vilib>:"DAQmx Clear Task.vi"("task in"=w414, "error in"=w413) -> ("error out"=w412:errorcluster)  [unwired: 13 out]
                n447 = case shown="False" "Sweep enabled" {
                  tunnel: [w455 w458] -> w437
                  tunnel: w430 -> [_ w457]
                  tunnel: w429 -> [w455 w456]
                  frame False {
                  }
                  frame True {
                    n448 = call <vilib>:"DAQmx Clear Task.vi"("task in"=w457, "error in"=w456) -> ("error out"=w458:errorcluster)  [unwired: 13 out]
                  }
                }
                n449 = Merge Errors(w447, w449, w412, w439, w440, w437) -> (w448:errorcluster)
                "error out" <- w448
                n450 = Transpose 2D Array(2D array=w352) -> (transposed array=w353:dbl[][])
                n451 = call <vilib>:"General Error Handler.vi"("error in (no error)"=w448) -> ()  [unwired: 10 in, 5 out]
                n452 = for {
                  tunnel: [w453] -> w340 mode=indexing
                  tunnel: w353 -> [w452] mode=indexing
                  n453 = call-poly <vilib>:"Basic Averaged DC-RMS.vi"("signal in"=w452) -> ("DC value"=w453:dbl)  [unwired: 7 in, 3 out]
                }
                n454 = To Single Precision Float(number=w340) -> (single precision float=w339:sgl[])
                n455 = Index Array(array=w339, index #1=0 ("index"), index #2=1 ("index"), index #3=2 ("index"), index #4=3 ("index"), index #5=4 ("index"), index #6=5 ("index")) -> (element #1=w342:sgl, element #2=w348:sgl, element #3=w347:sgl, element #4=w346:sgl, element #5=w345:sgl, element #6=w338:sgl)
                n456 = shared-variable ".\\Zeiss Library.lvlib\\Faraday cup offset"(w342) -> ()  [unwired: 1 in, 1 out]
                n457 = shared-variable ".\\Zeiss Library.lvlib\\Specimen (nA)"(w348) -> ()  [unwired: 1 in, 1 out]
                n458 = shared-variable ".\\Zeiss Library.lvlib\\Beam Dump 1 (nA)"(w347) -> ()  [unwired: 1 in, 1 out]
                n459 = shared-variable ".\\Zeiss Library.lvlib\\Beam Dump 2 (nA)"(w346) -> ()  [unwired: 1 in, 1 out]
                n460 = shared-variable ".\\Zeiss Library.lvlib\\Milling I (nA)"(w345) -> ()  [unwired: 1 in, 1 out]
                n461 = shared-variable ".\\Zeiss Library.lvlib\\Milling Z Voltage"(w338) -> ()  [unwired: 1 in, 1 out]
              }
              frame True {
                w761 = TRUE
              }
            }
          }
          frame #3 {
            n462 = local read "Sweep enabled"() -> (w762:bool)
            n463 = case shown="True" w762 {
              frame False {
              }
              frame True {
                n464 = local read "Post #1up"() -> (w767:tag)
                n465 = call-poly <vilib>:"DAQmx Create Virtual Channel.vi"("physical channels"=w767) -> ("task out"=w770:refnum<k21>, "error out"=w771:errorcluster)  [unwired: 13 in]
                n466 = local read "Post #1down"() -> (w766:tag)
                n467 = call-poly <vilib>:"DAQmx Create Virtual Channel.vi"("task in"=w770, "physical channels"=w766, "error in"=w771) -> ("task out"=w769:refnum<k21>, "error out"=w773:errorcluster)  [unwired: 11 in]
                n468 = local read "Post #2up"() -> (w764:tag)
                n469 = call-poly <vilib>:"DAQmx Create Virtual Channel.vi"("task in"=w769, "physical channels"=w764, "error in"=w773) -> ("task out"=w768:refnum<k21>, "error out"=w772:errorcluster)  [unwired: 11 in]
                n470 = local read "Post #2down"() -> (w765:tag)
                n471 = call-poly <vilib>:"DAQmx Create Virtual Channel.vi"("task in"=w768, "physical channels"=w765, "error in"=w772) -> ("task out"=w774:refnum<k21>, "error out"=w775:errorcluster)  [unwired: 11 in]
                n472 = call-poly <vilib>:"DAQmx Write.vi"("task/channels in"=w774, "data"=dbl[] [0.0, 0.0, 0.0, 0.0], "error in"=w775) -> ("task out"=w777:refnum<k21>, "error out"=w778:errorcluster)  [unwired: 1 in, 10 out]
                n473 = call <vilib>:"DAQmx Clear Task.vi"("task in"=w777, "error in"=w778) -> ("error out"=w763:errorcluster)  [unwired: 13 out]
                n474 = call <vilib>:"General Error Handler.vi"("error in (no error)"=w763) -> ()  [unwired: 10 in, 5 out]
                n475 = local write "error out"(w763) -> ()
              }
            }
          }
        }
        n476 = local read "Stop"() -> (w124:bool)
        n477 = Compound Arithmetic op=OR(w127, w131, w137, w124) -> (w128:bool)
      }
      n478 = case shown="True" w93 {
        frame False {
        }
        frame True {
          n479 = local write "Line Paused"(TRUE ("Line Paused")) -> ()
        }
      }
    }
    frame #2 {
      w781 = TRUE ("Beam blanked")
      n480 = local read "Machine Type"() -> (w780:u8)
      n481 = local read "Ext scan"() -> (w783:tag)
      n482 = local read "Beam blank"() -> (w785:tag)
      n483 = local write "Stop"(FALSE ("Stop")) -> ()
      n484 = local read "Api"() -> (w779:refnum<k7>)
      n485 = case shown="2" w780 {
        frame 0, Default {
        }
        frame 1 {
        }
        frame 2 {
          n486 = local read "Api"() -> (w790:refnum<k7>)
          n487 = call "SmartSEM Remote API set float.vi"("vValue"=sgl 2.0, "lpszParam"="DP_FIB_BLANKER_MODE" ("lpszCommand"), "Api"=w790) -> ("error out"=w786:errorcluster, "Api out"=w787:refnum<k7>)  [unwired: 7 in]
          n488 = call "SmartSEM Remote API FIB mode.vi"("error in"=w786, "FIB mode"=T5."SEM", "Api"=w787) -> ("error out"=w791:errorcluster, "Api out"=w792:refnum<k7>)  [unwired: 7 in]
          n489 = invoke class="_EMApi" method="Execute"(reference=w792, error in=w791, "lpszCommand"="CMD_FREEZE_ALL") -> ()  [unwired: 1 in, 4 out]
        }
      }
      n490 = local write "Beam blanked"(w781) -> ()
      n491 = call "FIB ext scan.vi"("Ext on"=FALSE ("data"), "FIB Ext Scan"=w783) -> ()  [unwired: 9 in, 1 out]
      n492 = call "FIB beam blank.vi"("Api"=w779, "Beam blanked"=w781, "lines"=w785) -> ()  [unwired: 2 in, 1 out]
    }
  }
